vi "Launch Two-Button Dialog Box.vi"(4 "Modal? (T)":bool=TRUE, 5 "False Button Return Message (Optional)":refnum<class "Abstract Dialog Return Msg.lvclass">, 7 "True Button Return Message (Optional)":refnum<class "Abstract Dialog Return Msg.lvclass">, 8 "False Button Text (Cancel)":string="Cancel", 9 "True Button Text (OK)":string="OK", 10 "Message Text":string, 11 "Dialog Launcher":refnum<class "IViewable.lvclass">) -> (0 "error out":errorcluster)   [LabVIEW 2015, in "TwoButtonDialogBox.lvlib" / "TwoButtonDialogBox.lvclass"]
uses:
  TwoButtonDialogBox.lvclass
  IViewable/IViewable/IViewable.lvclass
  IDialogBox/IDialogBox Abstract Messages/Abstract Dialog Return Msg/Abstract Dialog Return Msg.lvclass
  TwoButtonDialogBox.lvclass/TwoButtonDialogBox.ctl
  <vilib>/ActorFramework/Actor/Actor.lvclass/Actor.ctl
  <vilib>/ActorFramework/Message Enqueuer/Message Enqueuer.lvclass/Message Enqueuer.ctl
  IViewable/IViewable Messages/Launch Dialog Box Msg/Launch Dialog Box Msg.lvclass/Launch Dialog Box Msg.ctl
  <vilib>/ActorFramework/Message Enqueuer/Init from Existing Queue.vi
  <vilib>/ActorFramework/Message Enqueuer/Enqueue.vi
  <vilib>/ActorFramework/Message Priority Queue/Priority Enqueue.vi
  <vilib>/ActorFramework/Message Enqueuer/Message Enqueuer.lvclass
  IViewable/IViewable Messages/Launch Dialog Box Msg/Launch Dialog Box Msg.lvclass
  <vilib>/ActorFramework/Actor/Actor.lvclass
panel:
  in  "error in (no error)":errorcluster
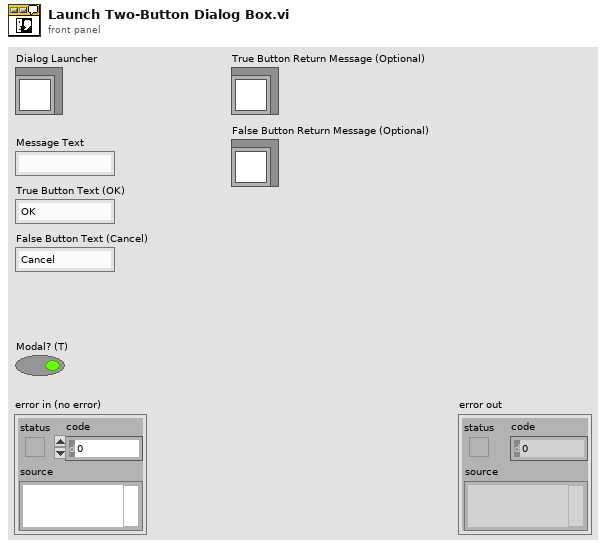
[diagram p1: front panel]
types:
  T1 = enum32{"Invalid", "Default", "Floating", "Floating/Auto-Hide", "Modal"}
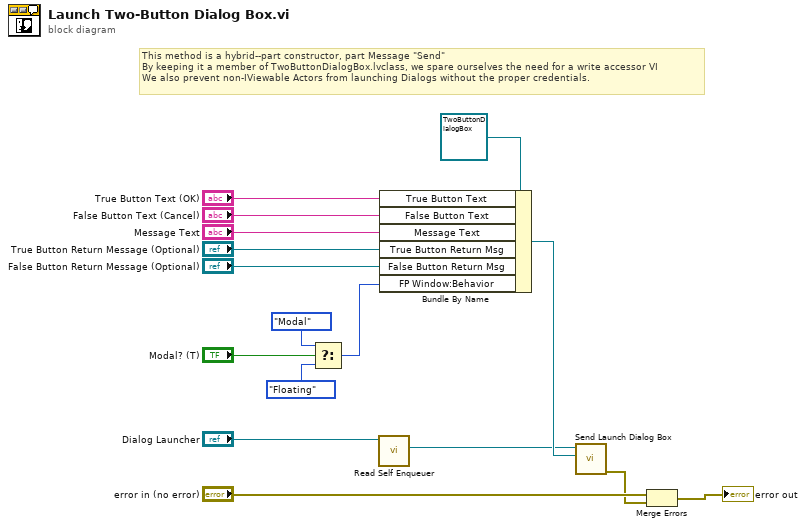
[diagram p0: block diagram]
diagram:
  # "This method is a hybrid--part constructor, part Message \"Send\"\nBy keeping it a member of TwoButtonDialogBox.lvclass, we spare ourselves the need for a write accessor VI\nWe also prevent non-IViewable Actors from launching Dialogs without the proper credentials."
  n1 = Select(t=T1."Modal" ("FP Window:Behavior"), s="Modal? (T)", f=T1."Floating" ("FP Window:Behavior")) -> (s? t:f=w3:T1)
  n2 = call <vilib>:"Read Self Enqueuer.vi"("Actor"="Dialog Launcher") -> ("Self Enqueuer"=w8:refnum<class "Message Enqueuer.lvclass">)  [unwired: 10 in]
  n3 = Bundle By Name(cluster=refnum<class "TwoButtonDialogBox.lvclass"> refnum ("OneButtonDialogBox in"), "True Button Text"="True Button Text (OK)", "False Button Text"="False Button Text (Cancel)", "Message Text"="Message Text", "True Button Return Msg"="True Button Return Message (Optional)", "False Button Return Msg"="False Button Return Message (Optional)", "FP Window:Behavior"=w3) -> (w11:refnum<class "TwoButtonDialogBox.lvclass">)
  n4 = call "Send Launch Dialog Box.vi"("DialogBox"=w11, "Message Enqueuer"=w8) -> ("error out"=w12:errorcluster)  [unwired: 8 in, 1 out]
  n5 = Merge Errors("error in (no error)", w12) -> (→"error out":errorcluster)
